vi "Lesson4 - Temperature Warnings subVI driver.vi"() -> ()   [LabVIEW 2013]
panel:
  out "Warning Text":string
  out "Warning?":bool
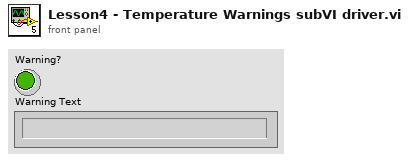
[diagram p1: front panel]
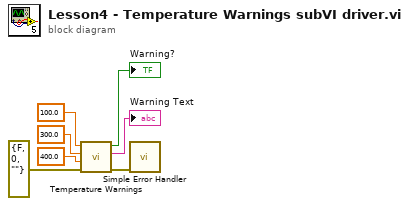
[diagram p0: block diagram]
diagram:
  n1 = call "Temperature Warnings.vi"("Error In"=errorcluster {"status"=FALSE, "code"=0, "source"=""}, "Min Temp"=400.0, "Max Temp"=300.0, "Current Temperature"=100.0) -> ("Error Out"=w3:errorcluster, "Warning Text"=→"Warning Text":string, "Warning?"=→"Warning?":bool)  [unwired: 3 in]
  n2 = call <vilib>:"Simple Error Handler.vi"("error in (no error)"=w3) -> ()  [unwired: 4 in, 5 out]
